vi "PID Lead-Lag (DBL Array).vi"(4 "reinitialize? (F)":bool, 5 "time unit":u16(ring)=1 items=["second", "minute"], 6 "dt (s)":dbl=-1.0 format="%.3f", 7 "output range":cluster{"output high":dbl, "output low":dbl}[](array[cluster])=[{"output high"=100.0, "output low"=-100.0}] {"output low" format="%.2f"; "output high" format="%.2f"}, 8 "tuning parameters":T1(array[cluster])=[{"gain"=1.0, "lag time"=0.01, "lead time"=0.0}] {"lead time" format="%.3f"; "lag time" format="%.3f"; "gain" format="%.3f"}, 9 "input":dbl[](array[numeric])=[0.0] format="%.2f") -> (0 "dt out (s)":dbl format="%.3f", 3 "output":dbl[](array[numeric]) format="%.2f")   [LabVIEW 2020, in "NI_PID_pid.lvlib"]
doc: "Implements a PID controller with a lead/lag function, which is generally used as a dynamic compensator in feedforward control schemes. This VI uses a positional algorithm and is an approximation of a true exponential lead/lag. Use the DBL instance of this VI to implement a single control loop. Use the DBL Array instance to implement parallel multi-loop control."
uses:
  <vilib>/addons/control/pid/NI_PID_pid.lvlib
panel:
  # "where:\nTlead: lead time\nTlag: lag time\nK: gain\nU(s): input\nY(s): output"
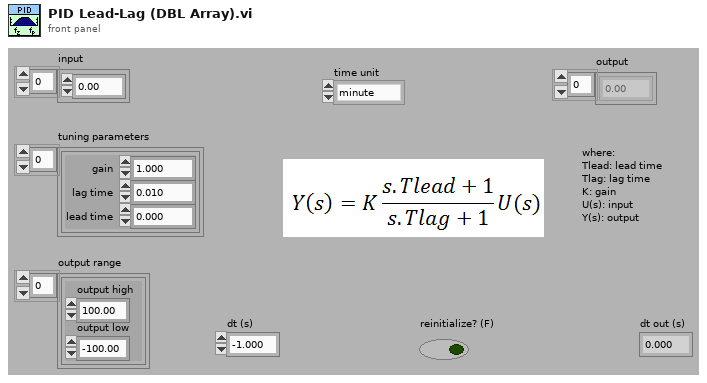
[diagram p1: front panel]
types:
  T1 = cluster{"gain":dbl, "lag time":dbl, "lead time":dbl}[]
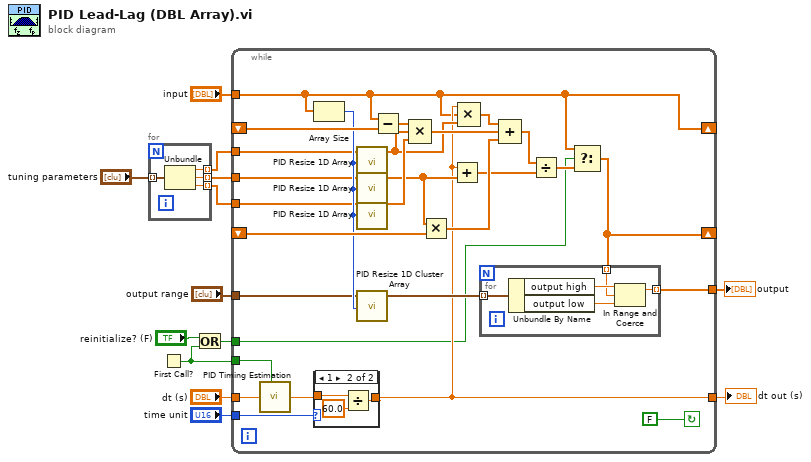
[diagram p0: block diagram]
diagram:
  n1 = for {
    tunnel: [w17] -> w5 mode=indexing
    tunnel: [w16] -> w7 mode=indexing
    tunnel: [w15] -> w6 mode=indexing
    tunnel: "tuning parameters" -> [w14] mode=indexing
    n2 = Unbundle(w14) -> ("gain"=w16:dbl, "lag time"=w15:dbl, "lead time"=w17:dbl)
  }
  n3 = First Call?() -> (First Call?: T/F=w10:bool)
  n4 = Or(x="reinitialize? (F)", y=w10) -> (x .or. y?=w12:bool)
  n5 = while {
    tunnel: w12 -> [w18]
    shift-left: _ -> [w43]
    shift-right: [w36] -> _
    shift-left: _ -> [w45]
    shift-right: [w22] -> _
    tunnel: "dt (s)" -> [w27]
    tunnel: w10 -> [w28]
    tunnel: [w26] -> w9
    tunnel: w7 -> [w25]
    tunnel: w6 -> [w24]
    tunnel: w5 -> [w23]
    tunnel: "input" -> [w22]
    tunnel: [w21] -> w3
    tunnel: "output range" -> [w20]
    tunnel: "time unit" -> [w19]
    stop <- FALSE continue-if-true
    n6 = call <vilib>:"PID Timing Estimation.vi"("Initialize?"=w28, "dt (s) in"=w27) -> ("dt (s) out"=w29:dbl)  [unwired: 7 in]
    n7 = Array Size(array=w22) -> (size(s)=w31:i32)
    n8 = case shown="1" w19 {
      tunnel: [w46 w48] -> w26
      tunnel: w29 -> [w46 w47]
      frame 0, Default {
      }
      frame 1 {
        n9 = Divide(x=w47, y=60.0) -> (x/y=w48:dbl)
      }
    }
    n10 = call <vilib>:"PID Resize 1D Array.vi"("array size"=w31, "input array"=w25) -> ("output array"=w33:dbl[])  [unwired: 3 out]
    n11 = call <vilib>:"PID Resize 1D Array.vi"("array size"=w31, "input array"=w24) -> ("output array"=w32:dbl[])  [unwired: 3 out]
    n12 = call <vilib>:"PID Resize 1D Array.vi"("array size"=w31, "input array"=w23) -> ("output array"=w34:dbl[])  [unwired: 3 out]
    n13 = call <vilib>:"PID Resize 1D Cluster Array.vi"("array size"=w31, "input array"=w20) -> ("output array"=w35:cluster{"output high":dbl, "output low":dbl}[])  [unwired: 3 out]
    n14 = Subtract(x=w22, y=w45) -> (x-y=w44:dbl[])
    n15 = Compound Arithmetic op=MULTIPLY(w44, w33, w34) -> (w41:dbl[])
    n16 = Multiply(x=w32, y=w43) -> (x*y=w40:dbl[])
    n17 = Add(x=w26, y=w32) -> (x+y=w38:dbl[])
    n18 = Compound Arithmetic op=MULTIPLY(w26, w22, w33) -> (w42:dbl[])
    n19 = Compound Arithmetic op=ADD(w42, w41, w40) -> (w39:dbl[])
    n20 = Divide(x=w39, y=w38) -> (x/y=w37:dbl[])
    n21 = Select(t=w22, s=w18, f=w37) -> (s? t:f=w36:dbl[])
    n22 = for {
      tunnel: w36 -> [w52] mode=indexing
      tunnel: w35 -> [w51] mode=indexing
      tunnel: [w50] -> w21 mode=indexing
      n23 = Unbundle By Name(w51) -> ("output high"=w54:dbl, "output low"=w53:dbl)
      n24 = In Range and Coerce(upper limit=w54, x=w52, lower limit=w53) -> (coerced(x)=w50:dbl)  [unwired: 1 out]
    }
  }
  "dt out (s)" <- w9
  "output" <- w3
